vi "set sensor mode.vi"(8 "error in (no error)":errorcluster, 11 "DAQOrcaFlash in":refnum<class "DAQOrcaFlash.lvclass">) -> (0 "error out":errorcluster, 3 "DAQOrcaFlash out":refnum<class "DAQOrcaFlash.lvclass">)   [LabVIEW 2012, in "DAQOrcaFlash.lvclass"]
uses:
  DAQOrcaFlash.lvclass
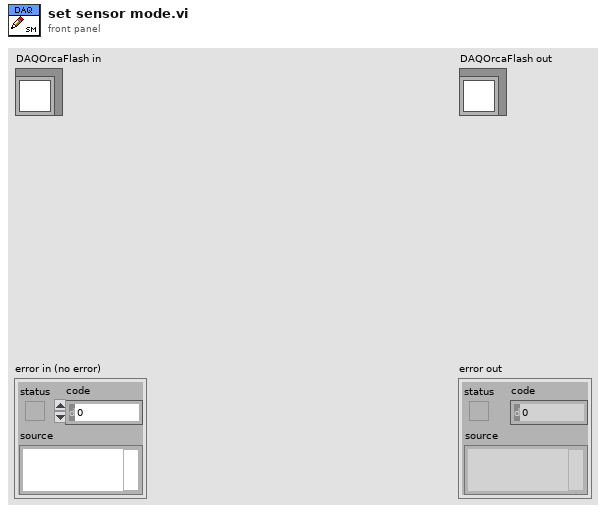
[diagram p1: front panel]
types:
  T1 = typedef "DAQOrcaFlash.lvclass/sensor_mode.ctl" = sgl
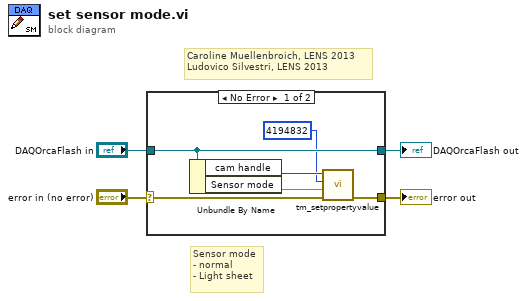
[diagram p0: block diagram]
diagram:
  # "Sensor mode\n- normal\n- Light sheet"
  # "Caroline Muellenbroich, LENS 2013\nLudovico Silvestri, LENS 2013"
  n1 = case shown="No Error" "error in (no error)" {
    selector: "error in (no error)" -> [w8 w12]
    tunnel: [w5 w12] -> w3
    tunnel: [w10 w11] -> w1
    tunnel: "DAQOrcaFlash in" -> [w10 w11]
    frame No Error {
      n2 = Unbundle By Name(w10) -> ("cam handle"=w9:u32, "Sensor mode"=w6:T1)
      n3 = call <userlib>:"tm_setpropertyvalue.vi"("error in (no error)"=w8, "Value in"=w6, "Property ID"=u32 4194832, "Handle in"=w9) -> ("error out"=w5:errorcluster)  [unwired: 6 in, 1 out]
    }
    frame Error {
    }
  }
  "error out" <- w3
  "DAQOrcaFlash out" <- w1
